vi "Configure TV Trigger Line Number [TV] Core.vi"(8 "error in (no error)":errorcluster, 10 "tv line number (1)":i32=1, 11 "CS++Scope":refnum<class "CS++Scope.lvclass">) -> (0 "error out":errorcluster, 3 "CS++Scope out":refnum<class "CS++Scope.lvclass">)   [LabVIEW 2013, in "CS++Scope.lvlib" / "CS++Scope.lvclass"]
doc: "This VI configures the TV line upon which the oscilloscope triggers. The line number is absolute and not relative to the field of the TV signal.\n\nNote\n\n(1) This VI affects instrument behavior only if the trigger type is set to\n IVISCOPE_VAL_TV_TRIGGER and the TV trigger event is set to\n IVISCOPE_VAL_TV_EVENT_LINE_NUMBER. Call the IviScope\n Configure Trigger and the IviScope Configure TV Trigger Source [TV]\n VIs to set the trigger type and TV trigger event before calling this VI\n.\n(2) This VI is part of the IviScopeTVTrigger [TV] extension group."
uses:
  CS++Scope.lvclass
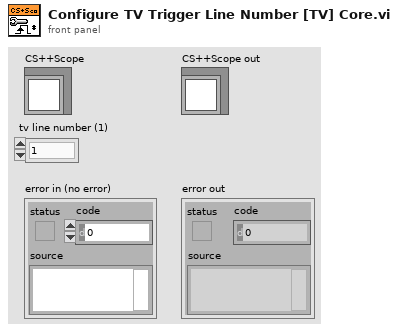
[diagram p1: front panel]
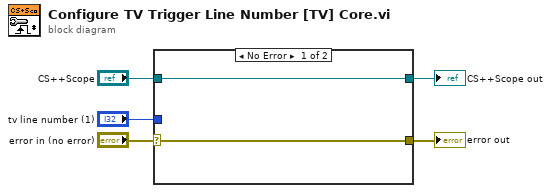
[diagram p0: block diagram]
diagram:
  n1 = case shown="No Error" "error in (no error)" {
    selector: "error in (no error)" -> [w6 w9]
    tunnel: [w6 w9] -> w4
    tunnel: [w7 w8] -> w2
    tunnel: "CS++Scope" -> [w7 w8]
    tunnel: "tv line number (1)" -> [_ _]
    frame No Error {
    }
    frame Error {
    }
  }
  "error out" <- w4
  "CS++Scope out" <- w2
